vi "Do Request.vi"(7 "Controller Inputs":T2, 8 "error in (no error)":errorcluster, 11 "File Upload Controller in":refnum<class "File Upload Controller.lvclass">) -> (0 "error out":errorcluster, 5 "Controller Outputs":T1)   [LabVIEW 2020, in "File Upload Controller.lvclass"]
uses:
  File Upload Controller.lvclass
  HTTP Server/Controller Inputs.ctl
  HTTP Server/Values/Values.lvclass
  <vilib>/IlluminatedG/IG HTTP Utils/HTTP Utils/Request/Request.lvclass
  HTTP Server/Session/Session.lvclass
  HTTP Server/Controller Outputs.ctl
  <vilib>/IlluminatedG/IG HTTP Utils/HTTP Utils/Response/Response.lvclass
  File Upload Controller.lvclass/File Upload Controller.ctl
  <vilib>/IlluminatedG/IG HTTP Utils/HTTP Utils/FormField/FormField.lvclass
  HTTP Server/HTTP Server.lvlib
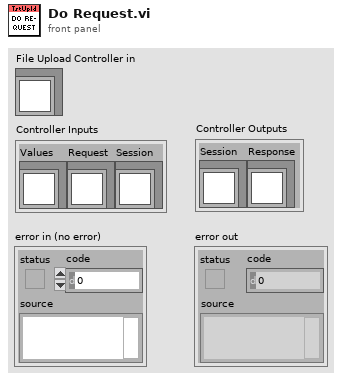
[diagram p1: front panel]
types:
  T1 = typedef "HTTP Server.lvlib/Controller Outputs.ctl" = cluster{"Session":refnum<class "Session.lvclass">, "Response":refnum<class "Response.lvclass">}
  T2 = typedef "HTTP Server.lvlib/Controller Inputs.ctl" = cluster{"Values":refnum<class "Values.lvclass">, "Request":refnum<class "Request.lvclass">, "Session":refnum<class "Session.lvclass">}
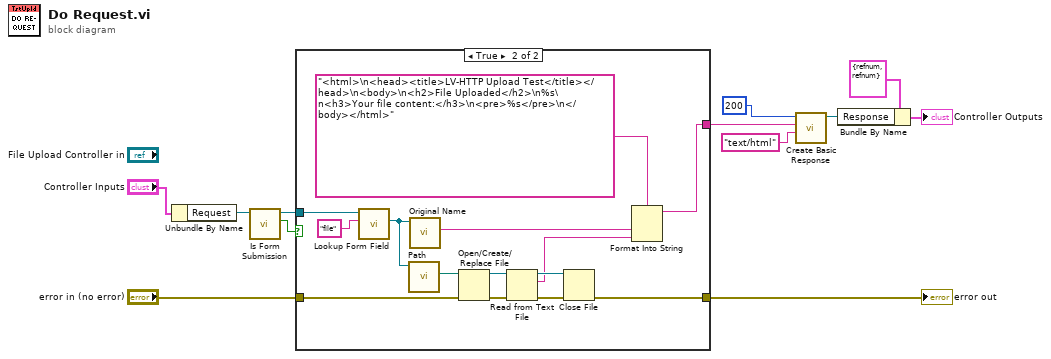
[diagram p0: block diagram]
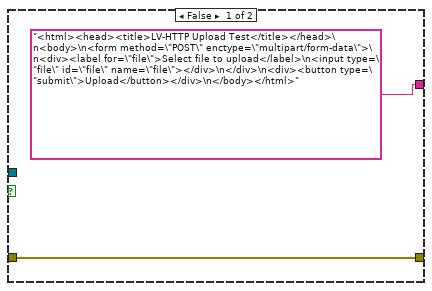
[diagram p2: hidden frame]
diagram:
  n1 = Unbundle By Name("Controller Inputs") -> ("Request"=w11:refnum<class "Request.lvclass">)
  n2 = call <vilib>:"Is Form Submission.vi"("Request in"=w11) -> ("Is Form Submission?"=w10:bool, "Request out"=w9:refnum<class "Request.lvclass">)  [unwired: 8 in, 1 out]
  n3 = case shown="True" w10 {
    tunnel: w9 -> [_ w28]
    tunnel: "error in (no error)" -> [w14 w23]
    tunnel: [w14 w19] -> w7
    tunnel: ["<html><head><title>LV-HTTP Upload Test</title></head>\n<body>\n<form method=\"POST\" enctype=\"multipart/form-data\">\n<div><label for=\"file\">Select file to upload</label>\n<input type=\"file\" id=\"file\" name=\"file\"></div>\n</div>\n<div><button type=\"submit\">Upload</button></div>\n</body></html>" w15] -> w6
    frame False {
    }
    frame True {
      n4 = call <vilib>:"Lookup Form Field.vi"("Name"="file", "Request in"=w28) -> ("Field"=w26:refnum<class "FormField.lvclass">)  [unwired: 6 in, 3 out]
      n5 = call <vilib>:"Path.vi"("FormField in"=w26) -> ("Path"=w25:path)  [unwired: 8 in, 2 out]
      n6 = call <vilib>:"Original Name.vi"("FormField in"=w26) -> ("Original Name"=w17:string)  [unwired: 8 in, 2 out]
      n7 = Open/Create/Replace File(file path (use dialog)=w25, error in=w23) -> (refnum out=w24:refnum<file>, error out=w22:errorcluster)  [unwired: 4 in, 1 out]
      n8 = Read from Text File(file (use dialog)=w24, error in=w22) -> (refnum out=w20:refnum<file>, text=w16:string, error out=w21:errorcluster)  [unwired: 2 in, 1 out]
      n9 = Close File(refnum=w20, error in=w21) -> (error out=w19:errorcluster)  [unwired: 1 out]
      n10 = Format Into String(format string="<html>\n<head><title>LV-HTTP Upload Test</title></head>\n<body>\n<h2>File Uploaded</h2>\n%s\n<h3>Your file content:</h3>\n<pre>%s</pre>\n</body></html>", w17, w16) -> (resulting string=w15:string)  [unwired: 2 in, 1 out]
    }
  }
  "error out" <- w7
  n11 = call <vilib>:"Create Basic Response.vi"("Content-Type (text/plain)"="text/html", "Payload"=w6, "Status Code"=u16 200) -> ("Response out"=w2:refnum<class "Response.lvclass">)  [unwired: 7 in, 1 out]
  n12 = Bundle By Name(cluster=T1 {"Session"=refnum, "Response"=refnum} ("Controller Outputs"), "Response"=w2) -> (→"Controller Outputs":T1)
